vi "del-group-eventSD.vi"(1 "cluster in":T1={"Kinetics"=[], "Spectrum"=[], "Experiments groups"=[], "GRAPH EXPERIMENTAL DATA"=[], "error out"={"status"=FALSE, "code"=0, "source"=""}, "group"=0, "exp selected"=0, "# exp"=0, "kinetics plot names"=[], "spectra plot names"=[], "FromToWave"={"FromWave"=0.0, "ToWave"=0.0}, "Laser shutter task"="", "Accelerator task"="", "Motor task"="", "GRAPH EXPERIMENTAL DATA ref"=refnum, "timedelays"=[0.0, 0.0, 0.0, 0.0, 0.0, 0.0, 0.0, 0.06019061100911815, 0.0521779104562645, 0.045231877429679615, 0.03921051490799832, 0.033990728811568754, 0.029465811603150715, 0.025543260876973825, 0.02214288834180205, 0.01919518054014414, 0.016639877791965713, 0.014424742312398925, 0.012504490320209958, 0.010839866306230088, 0.009396840537117498, 0.008145913389103785, 0.00706151229029317, 0.006121468943269439, 0.005306566140927374, 0.004600144911132549, 0.003987763959109073, 0.0034569044455719407, 0.00299671406541447, 0.0025977851951783253, 0.0022519625739982996, 0.00195217658646366, 0.0016922987392150965, 0.0014670163768006634, 0.0012717240756200802, 0.0011024294957352762, 0.0009556717658856477, 0.0008284507332614981, 0.0007181656316962257, 0.0006225619144775864, 0.0005396851648867825, 0.00046784114226338394, 0.0004055611468220084, 0.0003515719951773376, 0.00030476999279031153, 0.00026419837125694315, 0.00022902772919263772, 0.0001985390768670671, 0.0001721091379728629, 0.00014919760805372974, 0.00012933610911736794], "wavelengths"=[0.0, 0.0, 0.0, 0.0, 0.0, 0.0, 0.0, 0.06019061100911815, 0.0521779104562645, 0.045231877429679615, 0.03921051490799832, 0.033990728811568754, 0.029465811603150715, 0.025543260876973825, 0.02214288834180205, 0.01919518054014414, 0.016639877791965713, 0.014424742312398925, 0.012504490320209958, 0.010839866306230088, 0.009396840537117498, 0.008145913389103785, 0.00706151229029317, 0.006121468943269439, 0.005306566140927374, 0.004600144911132549, 0.003987763959109073, 0.0034569044455719407, 0.00299671406541447, 0.0025977851951783253, 0.0022519625739982996, 0.00195217658646366, 0.0016922987392150965, 0.0014670163768006634, 0.0012717240756200802, 0.0011024294957352762, 0.0009556717658856477, 0.0008284507332614981, 0.0007181656316962257, 0.0006225619144775864, 0.0005396851648867825, 0.00046784114226338394, 0.0004055611468220084, 0.0003515719951773376, 0.00030476999279031153, 0.00026419837125694315, 0.00022902772919263772, 0.0001985390768670671, 0.0001721091379728629, 0.00014919760805372974, 0.00012933610911736794], "Experiment"=refnum, "Commentaires exp"=refnum, "FromToDelay"={"FromDelay"=0.0, "ToDelay"=0.0}}, 2 "User Event in":refnum<user-event>) -> (0 "cluster out":T1={"Kinetics"=[], "Spectrum"=[], "Experiments groups"=[], "GRAPH EXPERIMENTAL DATA"=[], "error out"={"status"=FALSE, "code"=0, "source"=""}, "group"=0, "exp selected"=0, "# exp"=0, "kinetics plot names"=[], "spectra plot names"=[], "FromToWave"={"FromWave"=0.0, "ToWave"=0.0}, "Laser shutter task"="", "Accelerator task"="", "Motor task"="", "GRAPH EXPERIMENTAL DATA ref"=refnum, "timedelays"=[0.0, 0.0, 0.0, 0.0, 0.0, 0.0, 0.0, 0.06019061100911815, 0.0521779104562645, 0.045231877429679615, 0.03921051490799832, 0.033990728811568754, 0.029465811603150715, 0.025543260876973825, 0.02214288834180205, 0.01919518054014414, 0.016639877791965713, 0.014424742312398925, 0.012504490320209958, 0.010839866306230088, 0.009396840537117498, 0.008145913389103785, 0.00706151229029317, 0.006121468943269439, 0.005306566140927374, 0.004600144911132549, 0.003987763959109073, 0.0034569044455719407, 0.00299671406541447, 0.0025977851951783253, 0.0022519625739982996, 0.00195217658646366, 0.0016922987392150965, 0.0014670163768006634, 0.0012717240756200802, 0.0011024294957352762, 0.0009556717658856477, 0.0008284507332614981, 0.0007181656316962257, 0.0006225619144775864, 0.0005396851648867825, 0.00046784114226338394, 0.0004055611468220084, 0.0003515719951773376, 0.00030476999279031153, 0.00026419837125694315, 0.00022902772919263772, 0.0001985390768670671, 0.0001721091379728629, 0.00014919760805372974, 0.00012933610911736794], "wavelengths"=[0.0, 0.0, 0.0, 0.0, 0.0, 0.0, 0.0, 0.06019061100911815, 0.0521779104562645, 0.045231877429679615, 0.03921051490799832, 0.033990728811568754, 0.029465811603150715, 0.025543260876973825, 0.02214288834180205, 0.01919518054014414, 0.016639877791965713, 0.014424742312398925, 0.012504490320209958, 0.010839866306230088, 0.009396840537117498, 0.008145913389103785, 0.00706151229029317, 0.006121468943269439, 0.005306566140927374, 0.004600144911132549, 0.003987763959109073, 0.0034569044455719407, 0.00299671406541447, 0.0025977851951783253, 0.0022519625739982996, 0.00195217658646366, 0.0016922987392150965, 0.0014670163768006634, 0.0012717240756200802, 0.0011024294957352762, 0.0009556717658856477, 0.0008284507332614981, 0.0007181656316962257, 0.0006225619144775864, 0.0005396851648867825, 0.00046784114226338394, 0.0004055611468220084, 0.0003515719951773376, 0.00030476999279031153, 0.00026419837125694315, 0.00022902772919263772, 0.0001985390768670671, 0.0001721091379728629, 0.00014919760805372974, 0.00012933610911736794], "Experiment"=refnum, "Commentaires exp"=refnum, "FromToDelay"={"FromDelay"=0.0, "ToDelay"=0.0}})   [LabVIEW 2015]
uses:
  controls/control-cluster.ctl
  Classes/Experiments_group.lvclass
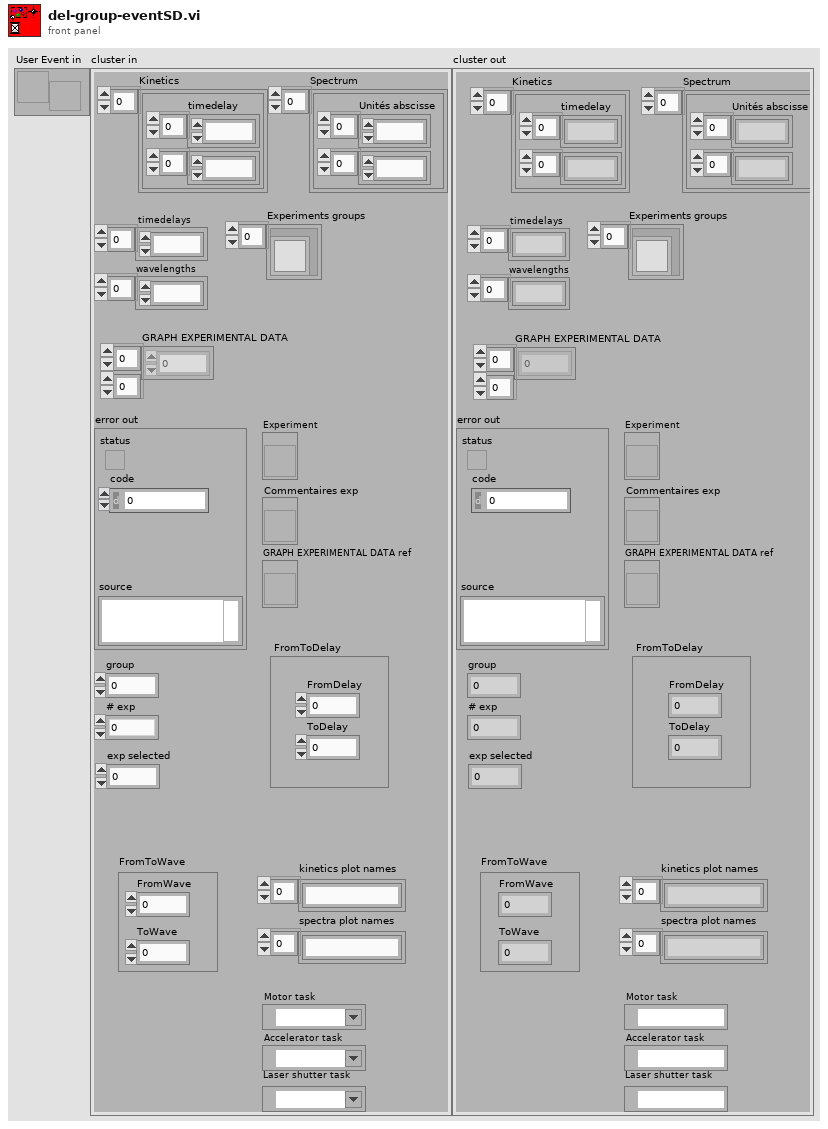
[diagram p1: front panel]
types:
  T1 = typedef "control-cluster.ctl" = cluster{"Kinetics":cluster{"timedelay":dbl[], dbl[]}[], "Spectrum":cluster{"Unités abscisse":dbl[], dbl[]}[], "Experiments groups":refnum<class "Experiments_group.lvclass">[], "GRAPH EXPERIMENTAL DATA":dbl[][], "error out":errorcluster, "group":i32, "exp selected":i32, "# exp":i32, "kinetics plot names":string[], "spectra plot names":string[], "FromToWave":cluster{"FromWave":dbl, "ToWave":dbl}, "Laser shutter task":refnum<k21>, "Accelerator task":refnum<k21>, "Motor task":refnum<k21>, "GRAPH EXPERIMENTAL DATA ref":refnum<vi>, "timedelays":dbl[], "wavelengths":dbl[], "Experiment":refnum<vi>, "Commentaires exp":refnum<vi>, "FromToDelay":cluster{"FromDelay":dbl, "ToDelay":dbl}}
  T2 = cluster{"Full/Part":bool, "Item names":string[], "Exp number":i32}
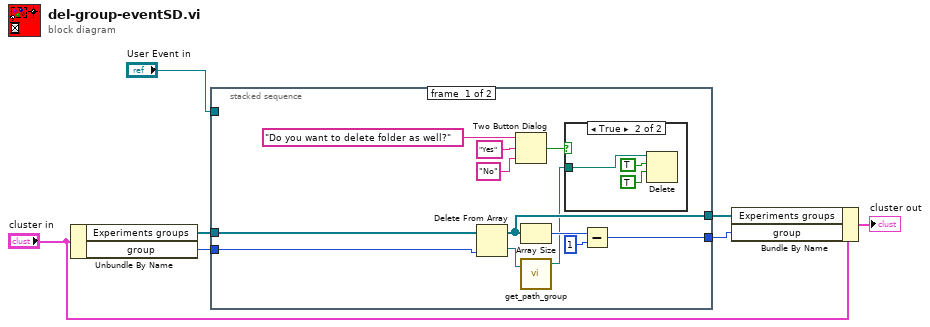
[diagram p0: block diagram]
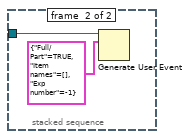
[diagram p3: hidden frame]
diagram:
  n1 = Unbundle By Name("cluster in") -> ("Experiments groups"=w4:refnum<class "Experiments_group.lvclass">[], "group"=w1:i32)
  n2 = stacked-sequence {
    tunnel: "User Event in" -> [_ w24]
    tunnel: w4 -> [w17 _]
    tunnel: [w16 _] -> w3
    tunnel: [w15 _] -> w2
    tunnel: w1 -> [w14 _]
    frame #0 {
      n3 = Delete From Array(array=w17, index=w14) -> (deleted portion=w13:refnum<class "Experiments_group.lvclass">, array with subset deleted=w16:refnum<class "Experiments_group.lvclass">[])  [unwired: 1 in]
      n4 = Two Button Dialog(message="Do you want to delete folder as well?", 1:"No" ("F button name (\"Cancel\")"), 2:"Yes" ("T button name (\"OK\")")) -> (T button?=w9:bool)
      n5 = Array Size(array=w16) -> (size(s)=w18:i32)
      n6 = call-dynamic "get_path_group.vi"("Experiments_group.lvclass in"=w13) -> ("Path"=w8:path)  [unwired: 1 in, 2 out]
      n7 = case shown="True" w9 {
        tunnel: w8 -> [_ w20]
        frame False {
        }
        frame True {
          n8 = Delete(path (use dialog)=w20, entire hierarchy (F)=TRUE, confirm (F)=TRUE) -> ()  [unwired: 2 in, 3 out]
        }
      }
      n9 = Subtract(x=w18, y=1) -> (x-y=w15:i32)
    }
    frame #1 {
      n10 = Generate User Event(user event=w24, event data cluster=T2 {"Full/Part"=TRUE, "Item names"=[], "Exp number"=-1} ("event data")) -> ()  [unwired: 2 in, 2 out]
    }
  }
  n11 = Bundle By Name(cluster="cluster in", "Experiments groups"=w3, "group"=w2) -> (→"cluster out":T1)
